vi "FPGA Target Approach Retraction2.vi"() -> ()   [LabVIEW 2012]
uses:
  <vilib>/rvi/interface/RandomDataEmulation/nirviRandomDataFPGAFIFO.vi
  <vilib>/rvi/interface/RandomDataEmulation/niFpgaRandomDataHandleErrors.vi
  <vilib>/rvi/eio/common/nirviEmuTemplateMethod_errors.vi
  <vilib>/rvi/DataTransferAndStorage/Container/XNode/niFpgaContainer.xnode
  <vilib>/rvi/interface/RandomDataEmulation/nirviRandomDataFpgaReadWriteTemplate.vi
  <vilib>/eio/EIONode/EIONode.xnode
  <vilib>/rvi/Analysis/measure/butterworth/XNode/niFpgaButterworthFilter.xnode
panel:
  out "Ticks":i16
  in  "Data Acquisition Rate":i16
  out "Tuning Fork Signal":fxp<+/-,24,17>
  out "HV/10":i16
  out "FPGA Output Voltage":fxp<+/-,64,32>
  out "Z Fine Indicator":fxp<+/-,40,30>
  out "Counter Indicator":i32
  in  "Z Fine Output":fxp<+/-,40,30>
  in  "Counter Output":i32
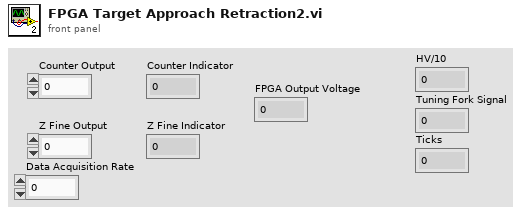
[diagram p1: front panel]
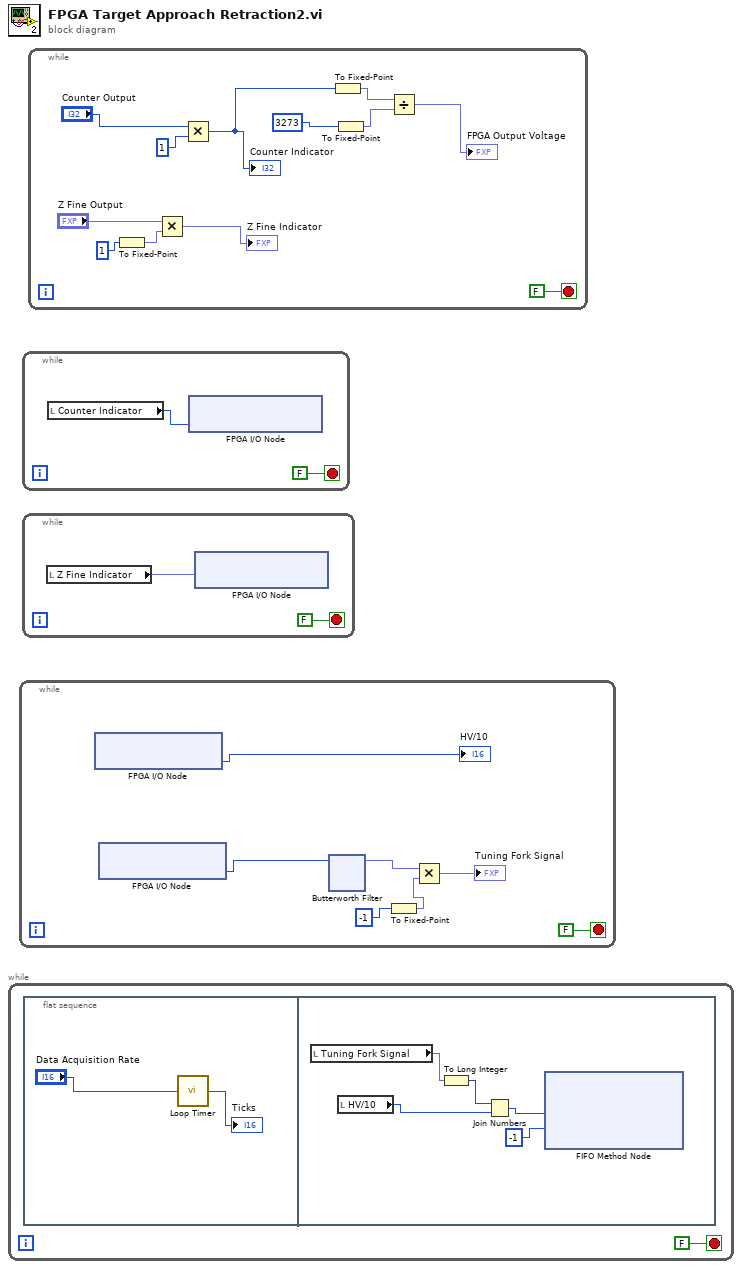
[diagram p0: block diagram]
diagram:
  n1 = while {
    stop <- FALSE stop-if-true
    n2 = flat-sequence {
      frame #0 {
        n3 = call "Loop Timer"("Count(uSec)"="Data Acquisition Rate") -> ("Tick Count(uSec)"=→"Ticks":u32)
      }
      frame #1 {
        n4 = local read "Tuning Fork Signal"() -> (w8:fxp<+/-,24,17>)
        n5 = local read "HV/10"() -> (w7:i16)
        n6 = To Long Integer(number=w8) -> (32bit integer=w6:i32)
        n7 = Join Numbers(hi=w6, lo=w7) -> ((hi.lo)=w5:u64)
        n8 = xnode ("FIFO Method Node")("Element"=w5, "Timeout"=i16 -1) -> ()  [unwired: 1 in, 2 out]
      }
    }
  }
  n9 = while {
    stop <- FALSE stop-if-true
    n10 = xnode "FPGA I/O Node"() -> ("Connector0/AI6"=→"HV/10":i16)  [unwired: 1 in, 1 out]
    n11 = xnode "FPGA I/O Node"() -> ("Connector0/AI7"=w14:i16)  [unwired: 1 in, 1 out]
    n12 = xnode "Butterworth Filter"("input data"=w14) -> ("output data"=w10:fxp<+/-,20,20>)  [unwired: 2 in]
    n13 = To Fixed-Point(number=i16 -1) -> (fixed-point=w11:fxp<+/-,16,16>)  [unwired: 1 in]
    n14 = Multiply(x=w10, y=w11) -> (x*y=→"Tuning Fork Signal":fxp<+/-,36,36>)
  }
  n15 = while {
    stop <- FALSE stop-if-true
    n16 = local read "Counter Indicator"() -> (w23:i32)
    n17 = xnode "FPGA I/O Node"("Connector0/AO7"=w23) -> ()  [unwired: 1 in, 1 out]
  }
  n18 = while {
    stop <- FALSE stop-if-true
    n19 = local read "Z Fine Indicator"() -> (w25:fxp<+/-,40,30>)
    n20 = xnode "FPGA I/O Node"("Connector0/AO2"=w25) -> ()  [unwired: 1 in, 1 out]
  }
  n21 = while {
    stop <- FALSE stop-if-true
    n22 = To Fixed-Point(number=1) -> (fixed-point=w33:fxp<+/-,32,32>)  [unwired: 1 in]
    n23 = Multiply(x="Z Fine Output", y=w33) -> (x*y=→"Z Fine Indicator":fxp<+/-,64,62>)
    n24 = Multiply(x="Counter Output", y=1) -> (x*y=w31:i32)
    "Counter Indicator" <- w31
    n25 = To Fixed-Point(number=w31) -> (fixed-point=w30:fxp<+/-,32,32>)  [unwired: 1 in]
    n26 = To Fixed-Point(number=3273) -> (fixed-point=w29:fxp<+/-,32,32>)  [unwired: 1 in]
    n27 = Divide(x=w30, y=w29) -> (x/y=→"FPGA Output Voltage":fxp<+/-,64,33>)
  }
